vi "Load Info.vi"(8 "error in":errorcluster, 11 "filename":path) -> (0 "error out":errorcluster, 3 "info data":string)   [LabVIEW 2019, in "infolib.lvlib"]
doc: "Reads whole info file. If filename not found, extension '.info' is added. If still no file found, error is generated."
uses:
  infolib.lvlib
  <vilib>/Utility/error.llb/Error Cluster From Error Code.vi
  <vilib>/ErrorRing/Error Ring.xnode
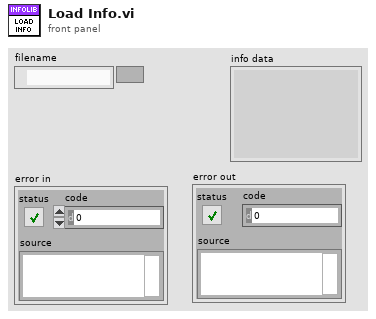
[diagram p1: front panel]
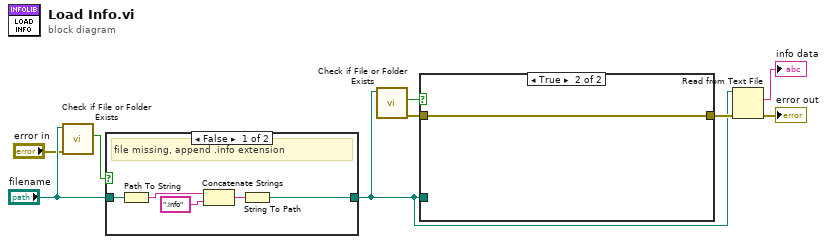
[diagram p0: block diagram]
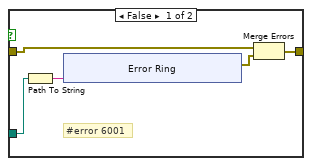
[diagram p3: hidden frame]
diagram:
  n1 = call <vilib>:"Check if File or Folder Exists.vi"("error in (no error)"="error in", "path"="filename") -> ("file or folder exists?"=w2:bool)  [unwired: 7 in, 2 out]
  n2 = case shown="False" w2 {
    tunnel: [w14 w15] -> w7
    tunnel: "filename" -> [w13 w15]
    frame False {
      # "file missing, append .info extension"
      n3 = Path To String(path=w13) -> (string=w11:string)
      n4 = Concatenate Strings(w11, ".info" ("y")) -> (w10:string)
      n5 = String To Path(string=w10) -> (path=w14:path)
    }
    frame True {
      # "file exist, do not append .info extension"
    }
  }
  n6 = call <vilib>:"Check if File or Folder Exists.vi"("path"=w7) -> ("error out"=w5:errorcluster, "file or folder exists?"=w6:bool)  [unwired: 8 in, 1 out]
  n7 = case shown="True" w6 {
    tunnel: w5 -> [w20 w28]
    tunnel: [w18 w28] -> w8
    tunnel: w7 -> [w16 _]
    frame False {
      # "#error 6001"
      n8 = Path To String(path=w16) -> (string=w17:string)
      n9 = xnode "Error Ring"("parameter 0"=w17) -> ("error out"=w19:errorcluster)
      n10 = Merge Errors(w20, w19) -> (w18:errorcluster)
    }
    frame True {
    }
  }
  n11 = Read from Text File(file (use dialog)=w7, error in=w8) -> (text=→"info data":string, error out=→"error out":errorcluster)  [unwired: 2 in, 2 out]
